vi "纳清_温度校准.vi"(7 "探头":T1(ring), 8 "error in (no error)":errorcluster caption="错误输入（无错误）", 10 "校准温度":sgl, 11 "MB session in":refnum<class "MB_Master.lvclass">) -> (0 "error out":errorcluster caption="错误输出", 3 "MB session out":refnum<class "MB_Master.lvclass">)   [LabVIEW 2016, in "斯坦道多参数.lvlib"]
uses:
  <vilib>/Plasmionique/MB Master/MB_Master/MB_Master.lvclass
  <vilib>/Plasmionique/MB Master/MB Master.lvlib
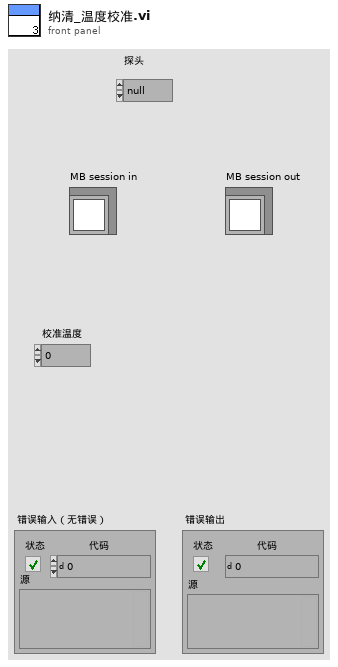
[diagram p1: front panel]
types:
  T1 = enum16{"null", "pH", "DO", "浊度", "电导率", "叶绿素a", "藻密度"}
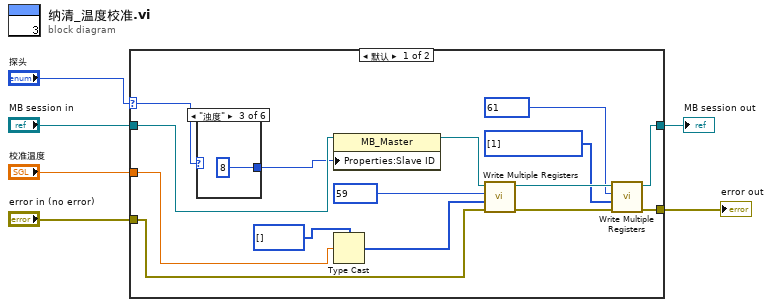
[diagram p0: block diagram]
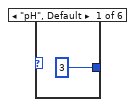
[diagram p2: hidden frame]
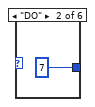
[diagram p3: hidden frame]
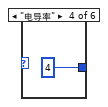
[diagram p4: hidden frame]
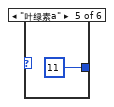
[diagram p5: hidden frame]
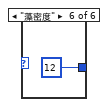
[diagram p6: hidden frame]
diagram:
  n1 = case shown="默认" "探头" {
    selector: "探头" -> [w14 _]
    tunnel: "error in (no error)" -> [w20 w28]
    tunnel: [w11 w28] -> w5
    tunnel: "MB session in" -> [w18 w29]
    tunnel: [w9 w29] -> w3
    tunnel: "校准温度" -> [w16 _]
    frame Default {
      n2 = case shown="\"浊度\"" w14 {
        tunnel: [3 7 8 4 11 12] -> w17
        frame "pH", Default {
        }
        frame "DO" {
        }
        frame "浊度" {
        }
        frame "电导率" {
        }
        frame "叶绿素a" {
        }
        frame "藻密度" {
        }
      }
      n3 = property class="MB_Master"(reference=w18, "Properties:Slave ID"=w17) -> (reference out=w19:refnum<class "MB_Master.lvclass">)  [unwired: 1 in, 1 out]
      n4 = Type Cast(type=u16[] [], x=w16) -> (*(type *) &x=w15:u16[])
      n5 = call <vilib>:"Write Multiple Registers.vi"("error in (no error)"=w20, "values"=w15, "starting address"=u16 59, "MB session in"=w19) -> ("error out"=w12:errorcluster, "MB session out"=w10:refnum<class "MB_Master.lvclass">)  [unwired: 6 in]
      n6 = call <vilib>:"Write Multiple Registers.vi"("error in (no error)"=w12, "values"=u16[] [1], "starting address"=u16 61, "MB session in"=w10) -> ("error out"=w11:errorcluster, "MB session out"=w9:refnum<class "MB_Master.lvclass">)  [unwired: 6 in]
    }
    frame "null" {
    }
  }
  "error out" <- w5
  "MB session out" <- w3
